vi "S4GUI.vi"(7 "Tab ObsEng":enum32{"Obs", "CCD modes", "Guider", "Eng"}(tab)) -> ()   [LabVIEW 2018] (continued)
                    n4631 = invoke class="VI" method="Run VI"(reference=w10986, error in=w10987, "Wait until done"=w10984, "Auto Dispose Ref"=w10984) -> ()  [unwired: 1 in, 5 out]
                  }
                }
              }
            }
            n4632 = Number To Decimal String(number="Target Temp 4") -> (decimal integer string=w10906:string)  [unwired: 1 in]
            n4633 = call-dynamic "Write Channel.vi"("error in (no error)"=w10889, "Channel.lvclass"=w10892, "Acquisition in"=w10891) -> ("error out"=w10922:errorcluster, "Acquisition out"=w10923:refnum<class "Acquisition.lvclass">)  [unwired: 7 in]
            n4634 = Concatenate Strings("SET TEMP [" ("User Event"), w10906, "] CLICKED - CH4" ("User Event")) -> (w10905:string)
            n4635 = call-dynamic "Write AcquisitionD.vi"("error in (no error)"=w10922, "Acquisition.lvclass"=w10923, "S4ACS_GUI in"=w10890) -> ("error out"=w10900:errorcluster, "S4ACS_GUI out"=w10901:refnum<class "S4GUI.lvclass">)  [unwired: 7 in]
            n4636 = call-dynamic "Write User Event.vi"("error in (no error)"=w10900, "User Event"=w10905, "S4GUI in"=w10901) -> ("error out"=w10898:errorcluster, "S4GUI out"=w10899:refnum<class "S4GUI.lvclass">)  [unwired: 7 in]
          }
        }
      }
      event "SET Temp message": Value Change {
        # "Seleção do modo de apresentação da\nmensagem de erro para o SET de \ntemperatura manual:\nF: via Last Error em vermelho (S4GUI:HandleObservation.vi);\nT: via janela de popup (MsgTempPopup.vi)."
        n4637 = event-data() -> ("NewVal"=w10993:bool)  [unwired: 1 in]
        n4638 = call-dynamic "Write SET temp error mode.vi"("error in (no error)"=w10994, "SET temp error mode"=w10993, "S4GUI in"=w10995) -> ("error out"=w10991:errorcluster, "S4GUI out"=w10992:refnum<class "S4GUI.lvclass">)  [unwired: 7 in]
      }
      event "Avança Estado": Value Change {
        n4639 = event-data() -> ()  [unwired: 1 in, 4 out]
        n4640 = call-dynamic "Read Sync Box.lvclass.vi"("error in (no error)"=w11004, "SPARC4_AC in"=w11005) -> ("error out"=w11017:errorcluster, "Sync Box.lvclass"=w11018:refnum<class "Sync Box.lvclass">, "SPARC4_AC out"=w11009:refnum<class "S4GUI.lvclass">)  [unwired: 7 in]
        n4641 = call-dynamic "Read Trigger.lvclass.vi"("error in (no error)"=w11017, "Sync Box in"=w11018) -> ("error out"=w11015:errorcluster, "Trigger.lvclass"=w11016:refnum<class "Trigger.lvclass">, "Sync Box out"=w11012:refnum<class "Sync Box.lvclass">)  [unwired: 7 in]
        n4642 = call-dynamic "Read State Machine.vi"("error in (no error)"=w11015, "Device in"=w11016) -> ("error out"=w11001:errorcluster, "State Machine.lvclass"=w11002:refnum<class "State Machine.lvclass">, "Device out"=w11013:refnum<class "Trigger.lvclass">)  [unwired: 7 in]
        n4643 = call-dynamic "Read State.vi"("error in (no error)"=w11001, "State Machine in"=w11002) -> ("error out"=w10997:errorcluster, "State"=w11000:i32, "State Machine out"=w10998:refnum<class "State Machine.lvclass">)  [unwired: 7 in]
        n4644 = Increment(x=w11000) -> (x+1=w10999:i32)
        n4645 = call "Next State.vi"("error in (no error)"=w10997, "New_State"=w10999, "State Machine in"=w10998) -> ("error out"=w11011:errorcluster, "State Machine out"=w11014:refnum<class "State Machine.lvclass">)  [unwired: 7 in]
        n4646 = call-dynamic "Write State Machine.vi"("error in (no error)"=w11011, "State Machine.lvclass"=w11014, "Device in"=w11013) -> ("error out"=w11007:errorcluster, "Device out"=w11006:refnum<class "Trigger.lvclass">)  [unwired: 7 in]
        n4647 = call-dynamic "Write Trigger.lvclass.vi"("error in (no error)"=w11007, "Trigger.lvclass"=w11006, "Sync Box in"=w11012) -> ("error out"=w11008:errorcluster, "Sync Box out"=w11010:refnum<class "Sync Box.lvclass">)  [unwired: 7 in]
        n4648 = call-dynamic "Write Sync Box.lvclass.vi"("error in (no error)"=w11008, "Sync Box.lvclass"=w11010, "SPARC4_AC in"=w11009) -> ("error out"=w11003:errorcluster, "SPARC4_AC out"=w10996:refnum<class "S4GUI.lvclass">)  [unwired: 7 in]
      }
      event "DelayA": Value Change {
        n4649 = event-data() -> ("NewVal"=w11020:string)  [unwired: 1 in, 3 out]
        n4650 = call-dynamic "Read Sync Box.lvclass.vi"("error in (no error)"=w11024, "SPARC4_AC in"=w11025) -> ("error out"=w11032:errorcluster, "Sync Box.lvclass"=w11033:refnum<class "Sync Box.lvclass">, "SPARC4_AC out"=w11029:refnum<class "S4GUI.lvclass">)  [unwired: 7 in]
        n4651 = call-dynamic "Read Trigger.lvclass.vi"("error in (no error)"=w11032, "Sync Box in"=w11033) -> ("error out"=w11021:errorcluster, "Trigger.lvclass"=w11022:refnum<class "Trigger.lvclass">, "Sync Box out"=w11031:refnum<class "Sync Box.lvclass">)  [unwired: 7 in]
        n4652 = call-dynamic "Write DelayA.vi"("error in (no error)"=w11021, "DelayA"=w11020, "Trigger in"=w11022) -> ("error out"=w11027:errorcluster, "Trigger out"=w11026:refnum<class "Trigger.lvclass">)  [unwired: 7 in]
        n4653 = call-dynamic "Write Trigger.lvclass.vi"("error in (no error)"=w11027, "Trigger.lvclass"=w11026, "Sync Box in"=w11031) -> ("error out"=w11028:errorcluster, "Sync Box out"=w11030:refnum<class "Sync Box.lvclass">)  [unwired: 7 in]
        n4654 = call-dynamic "Write Sync Box.lvclass.vi"("error in (no error)"=w11028, "Sync Box.lvclass"=w11030, "SPARC4_AC in"=w11029) -> ("error out"=w11023:errorcluster, "SPARC4_AC out"=w11019:refnum<class "S4GUI.lvclass">)  [unwired: 7 in]
      }
      event "DelayB": Value Change {
        n4655 = event-data() -> ("NewVal"=w11035:string)  [unwired: 1 in, 3 out]
        n4656 = call-dynamic "Read Sync Box.lvclass.vi"("error in (no error)"=w11039, "SPARC4_AC in"=w11040) -> ("error out"=w11047:errorcluster, "Sync Box.lvclass"=w11048:refnum<class "Sync Box.lvclass">, "SPARC4_AC out"=w11044:refnum<class "S4GUI.lvclass">)  [unwired: 7 in]
        n4657 = call-dynamic "Read Trigger.lvclass.vi"("error in (no error)"=w11047, "Sync Box in"=w11048) -> ("error out"=w11036:errorcluster, "Trigger.lvclass"=w11037:refnum<class "Trigger.lvclass">, "Sync Box out"=w11046:refnum<class "Sync Box.lvclass">)  [unwired: 7 in]
        n4658 = call-dynamic "Write DelayB.vi"("error in (no error)"=w11036, "DelayB"=w11035, "Trigger in"=w11037) -> ("error out"=w11042:errorcluster, "Trigger out"=w11041:refnum<class "Trigger.lvclass">)  [unwired: 7 in]
        n4659 = call-dynamic "Write Trigger.lvclass.vi"("error in (no error)"=w11042, "Trigger.lvclass"=w11041, "Sync Box in"=w11046) -> ("error out"=w11043:errorcluster, "Sync Box out"=w11045:refnum<class "Sync Box.lvclass">)  [unwired: 7 in]
        n4660 = call-dynamic "Write Sync Box.lvclass.vi"("error in (no error)"=w11043, "Sync Box.lvclass"=w11045, "SPARC4_AC in"=w11044) -> ("error out"=w11038:errorcluster, "SPARC4_AC out"=w11034:refnum<class "S4GUI.lvclass">)  [unwired: 7 in]
      }
      event "DelayC": Value Change {
        n4661 = event-data() -> ("NewVal"=w11050:string)  [unwired: 1 in, 3 out]
        n4662 = call-dynamic "Read Sync Box.lvclass.vi"("error in (no error)"=w11054, "SPARC4_AC in"=w11055) -> ("error out"=w11062:errorcluster, "Sync Box.lvclass"=w11063:refnum<class "Sync Box.lvclass">, "SPARC4_AC out"=w11059:refnum<class "S4GUI.lvclass">)  [unwired: 7 in]
        n4663 = call-dynamic "Read Trigger.lvclass.vi"("error in (no error)"=w11062, "Sync Box in"=w11063) -> ("error out"=w11051:errorcluster, "Trigger.lvclass"=w11052:refnum<class "Trigger.lvclass">, "Sync Box out"=w11061:refnum<class "Sync Box.lvclass">)  [unwired: 7 in]
        n4664 = call-dynamic "Write DelayC.vi"("error in (no error)"=w11051, "DelayC"=w11050, "Trigger in"=w11052) -> ("error out"=w11057:errorcluster, "Trigger out"=w11056:refnum<class "Trigger.lvclass">)  [unwired: 7 in]
        n4665 = call-dynamic "Write Trigger.lvclass.vi"("error in (no error)"=w11057, "Trigger.lvclass"=w11056, "Sync Box in"=w11061) -> ("error out"=w11058:errorcluster, "Sync Box out"=w11060:refnum<class "Sync Box.lvclass">)  [unwired: 7 in]
        n4666 = call-dynamic "Write Sync Box.lvclass.vi"("error in (no error)"=w11058, "Sync Box.lvclass"=w11060, "SPARC4_AC in"=w11059) -> ("error out"=w11053:errorcluster, "SPARC4_AC out"=w11049:refnum<class "S4GUI.lvclass">)  [unwired: 7 in]
      }
      event "DelayD": Value Change {
        n4667 = event-data() -> ("NewVal"=w11065:string)  [unwired: 1 in, 3 out]
        n4668 = call-dynamic "Read Sync Box.lvclass.vi"("error in (no error)"=w11069, "SPARC4_AC in"=w11070) -> ("error out"=w11077:errorcluster, "Sync Box.lvclass"=w11078:refnum<class "Sync Box.lvclass">, "SPARC4_AC out"=w11074:refnum<class "S4GUI.lvclass">)  [unwired: 7 in]
        n4669 = call-dynamic "Read Trigger.lvclass.vi"("error in (no error)"=w11077, "Sync Box in"=w11078) -> ("error out"=w11066:errorcluster, "Trigger.lvclass"=w11067:refnum<class "Trigger.lvclass">, "Sync Box out"=w11076:refnum<class "Sync Box.lvclass">)  [unwired: 7 in]
        n4670 = call-dynamic "Write DelayD.vi"("error in (no error)"=w11066, "DelayD"=w11065, "Trigger in"=w11067) -> ("error out"=w11072:errorcluster, "Trigger out"=w11071:refnum<class "Trigger.lvclass">)  [unwired: 7 in]
        n4671 = call-dynamic "Write Trigger.lvclass.vi"("error in (no error)"=w11072, "Trigger.lvclass"=w11071, "Sync Box in"=w11076) -> ("error out"=w11073:errorcluster, "Sync Box out"=w11075:refnum<class "Sync Box.lvclass">)  [unwired: 7 in]
        n4672 = call-dynamic "Write Sync Box.lvclass.vi"("error in (no error)"=w11073, "Sync Box.lvclass"=w11075, "SPARC4_AC in"=w11074) -> ("error out"=w11068:errorcluster, "SPARC4_AC out"=w11064:refnum<class "S4GUI.lvclass">)  [unwired: 7 in]
      }
      event "WidthA": Value Change {
        n4673 = event-data() -> ("NewVal"=w11080:string)  [unwired: 1 in, 3 out]
        n4674 = call-dynamic "Read Sync Box.lvclass.vi"("error in (no error)"=w11084, "SPARC4_AC in"=w11085) -> ("error out"=w11092:errorcluster, "Sync Box.lvclass"=w11093:refnum<class "Sync Box.lvclass">, "SPARC4_AC out"=w11089:refnum<class "S4GUI.lvclass">)  [unwired: 7 in]
        n4675 = call-dynamic "Read Trigger.lvclass.vi"("error in (no error)"=w11092, "Sync Box in"=w11093) -> ("error out"=w11081:errorcluster, "Trigger.lvclass"=w11082:refnum<class "Trigger.lvclass">, "Sync Box out"=w11091:refnum<class "Sync Box.lvclass">)  [unwired: 7 in]
        n4676 = call-dynamic "Write WidthA.vi"("error in (no error)"=w11081, "WidthA"=w11080, "Trigger in"=w11082) -> ("error out"=w11087:errorcluster, "Trigger out"=w11086:refnum<class "Trigger.lvclass">)  [unwired: 7 in]
        n4677 = call-dynamic "Write Trigger.lvclass.vi"("error in (no error)"=w11087, "Trigger.lvclass"=w11086, "Sync Box in"=w11091) -> ("error out"=w11088:errorcluster, "Sync Box out"=w11090:refnum<class "Sync Box.lvclass">)  [unwired: 7 in]
        n4678 = call-dynamic "Write Sync Box.lvclass.vi"("error in (no error)"=w11088, "Sync Box.lvclass"=w11090, "SPARC4_AC in"=w11089) -> ("error out"=w11083:errorcluster, "SPARC4_AC out"=w11079:refnum<class "S4GUI.lvclass">)  [unwired: 7 in]
      }
      event "WidthB": Value Change {
        n4679 = event-data() -> ("NewVal"=w11095:string)  [unwired: 1 in, 3 out]
        n4680 = call-dynamic "Read Sync Box.lvclass.vi"("error in (no error)"=w11099, "SPARC4_AC in"=w11100) -> ("error out"=w11107:errorcluster, "Sync Box.lvclass"=w11108:refnum<class "Sync Box.lvclass">, "SPARC4_AC out"=w11104:refnum<class "S4GUI.lvclass">)  [unwired: 7 in]
        n4681 = call-dynamic "Read Trigger.lvclass.vi"("error in (no error)"=w11107, "Sync Box in"=w11108) -> ("error out"=w11096:errorcluster, "Trigger.lvclass"=w11097:refnum<class "Trigger.lvclass">, "Sync Box out"=w11106:refnum<class "Sync Box.lvclass">)  [unwired: 7 in]
        n4682 = call-dynamic "Write WidthB.vi"("error in (no error)"=w11096, "WidthB"=w11095, "Trigger in"=w11097) -> ("error out"=w11102:errorcluster, "Trigger out"=w11101:refnum<class "Trigger.lvclass">)  [unwired: 7 in]
        n4683 = call-dynamic "Write Trigger.lvclass.vi"("error in (no error)"=w11102, "Trigger.lvclass"=w11101, "Sync Box in"=w11106) -> ("error out"=w11103:errorcluster, "Sync Box out"=w11105:refnum<class "Sync Box.lvclass">)  [unwired: 7 in]
        n4684 = call-dynamic "Write Sync Box.lvclass.vi"("error in (no error)"=w11103, "Sync Box.lvclass"=w11105, "SPARC4_AC in"=w11104) -> ("error out"=w11098:errorcluster, "SPARC4_AC out"=w11094:refnum<class "S4GUI.lvclass">)  [unwired: 7 in]
      }
      event "WidthC": Value Change {
        n4685 = event-data() -> ("NewVal"=w11110:string)  [unwired: 1 in, 3 out]
        n4686 = call-dynamic "Read Sync Box.lvclass.vi"("error in (no error)"=w11114, "SPARC4_AC in"=w11115) -> ("error out"=w11122:errorcluster, "Sync Box.lvclass"=w11123:refnum<class "Sync Box.lvclass">, "SPARC4_AC out"=w11119:refnum<class "S4GUI.lvclass">)  [unwired: 7 in]
        n4687 = call-dynamic "Read Trigger.lvclass.vi"("error in (no error)"=w11122, "Sync Box in"=w11123) -> ("error out"=w11111:errorcluster, "Trigger.lvclass"=w11112:refnum<class "Trigger.lvclass">, "Sync Box out"=w11121:refnum<class "Sync Box.lvclass">)  [unwired: 7 in]
        n4688 = call-dynamic "Write WidthC.vi"("error in (no error)"=w11111, "WidthC"=w11110, "Trigger in"=w11112) -> ("error out"=w11117:errorcluster, "Trigger out"=w11116:refnum<class "Trigger.lvclass">)  [unwired: 7 in]
        n4689 = call-dynamic "Write Trigger.lvclass.vi"("error in (no error)"=w11117, "Trigger.lvclass"=w11116, "Sync Box in"=w11121) -> ("error out"=w11118:errorcluster, "Sync Box out"=w11120:refnum<class "Sync Box.lvclass">)  [unwired: 7 in]
        n4690 = call-dynamic "Write Sync Box.lvclass.vi"("error in (no error)"=w11118, "Sync Box.lvclass"=w11120, "SPARC4_AC in"=w11119) -> ("error out"=w11113:errorcluster, "SPARC4_AC out"=w11109:refnum<class "S4GUI.lvclass">)  [unwired: 7 in]
      }
      event "WidthD": Value Change {
        n4691 = event-data() -> ("NewVal"=w11125:string)  [unwired: 1 in, 3 out]
        n4692 = call-dynamic "Read Sync Box.lvclass.vi"("error in (no error)"=w11129, "SPARC4_AC in"=w11130) -> ("error out"=w11137:errorcluster, "Sync Box.lvclass"=w11138:refnum<class "Sync Box.lvclass">, "SPARC4_AC out"=w11134:refnum<class "S4GUI.lvclass">)  [unwired: 7 in]
        n4693 = call-dynamic "Read Trigger.lvclass.vi"("error in (no error)"=w11137, "Sync Box in"=w11138) -> ("error out"=w11126:errorcluster, "Trigger.lvclass"=w11127:refnum<class "Trigger.lvclass">, "Sync Box out"=w11136:refnum<class "Sync Box.lvclass">)  [unwired: 7 in]
        n4694 = call-dynamic "Write WidthD.vi"("error in (no error)"=w11126, "WidthD"=w11125, "Trigger in"=w11127) -> ("error out"=w11132:errorcluster, "Trigger out"=w11131:refnum<class "Trigger.lvclass">)  [unwired: 7 in]
        n4695 = call-dynamic "Write Trigger.lvclass.vi"("error in (no error)"=w11132, "Trigger.lvclass"=w11131, "Sync Box in"=w11136) -> ("error out"=w11133:errorcluster, "Sync Box out"=w11135:refnum<class "Sync Box.lvclass">)  [unwired: 7 in]
        n4696 = call-dynamic "Write Sync Box.lvclass.vi"("error in (no error)"=w11133, "Sync Box.lvclass"=w11135, "SPARC4_AC in"=w11134) -> ("error out"=w11128:errorcluster, "SPARC4_AC out"=w11124:refnum<class "S4GUI.lvclass">)  [unwired: 7 in]
      }
      event "WPROT_set": Value Change {
        # "Espera até 10 x 1s = 10s\npara condition de WPROT\n ir para READY"
        n4697 = event-data() -> ()  [unwired: 1 in, 4 out]
        n4698 = call "Read Instrument.lvclass.vi"("error in (no error)"=w11160, "S4ACS_GUI in"=w11161) -> ("error out"=w11158:errorcluster, "Instrument.lvclass"=w11159:refnum<class "Instrument.lvclass">, "S4ACS_GUI out"=w11147:refnum<class "S4GUI.lvclass">)  [unwired: 7 in]
        n4699 = call "Read WPROT.vi"("error in (no error)"=w11158, "Instrument in"=w11159) -> ("error out"=w11154:errorcluster, "Opt_Selector.lvclass"=w11157:refnum<class "Opt_Selector.lvclass">, "Instrument out"=w11150:refnum<class "Instrument.lvclass">)  [unwired: 7 in]
        n4700 = call-dynamic "Read State Machine.vi"("error in (no error)"=w11154, "Device in"=w11157) -> ("error out"=w11153:errorcluster, "State Machine.lvclass"=w11156:refnum<class "State Machine.lvclass">, "Device out"=w11152:refnum<class "Opt_Selector.lvclass">)  [unwired: 7 in]
        n4701 = call "Next State.vi"("error in (no error)"=w11153, "New_State"=1, "State Machine in"=w11156) -> ("error out"=w11141:errorcluster, "State Machine out"=w11143:refnum<class "State Machine.lvclass">)  [unwired: 7 in]
        n4702 = call-dynamic "Write Timer.vi"("error in (no error)"=w11141, "Timer"=u32 10, "State Machine in"=w11143) -> ("error out"=w11140:errorcluster, "State Machine out"=w11142:refnum<class "State Machine.lvclass">)  [unwired: 7 in]
        n4703 = call-dynamic "Write State Machine.vi"("error in (no error)"=w11140, "State Machine.lvclass"=w11142, "Device in"=w11152) -> ("error out"=w11149:errorcluster, "Device out"=w11151:refnum<class "Opt_Selector.lvclass">)  [unwired: 7 in]
        n4704 = call "Write WPROT.vi"("error in (no error)"=w11149, "Opt_Selector.lvclass"=w11151, "Instrument in"=w11150) -> ("error out"=w11146:errorcluster, "Instrument out"=w11148:refnum<class "Instrument.lvclass">)  [unwired: 7 in]
        n4705 = call "Write Instrument.lvclass.vi"("error in (no error)"=w11146, "Instrument.lvclass"=w11148, "S4ACS_GUI in"=w11147) -> ("error out"=w11145:errorcluster, "S4ACS_GUI out"=w11144:refnum<class "S4GUI.lvclass">)  [unwired: 7 in]
      }
      event "TARGET NAME WPROT": Value Change {
        n4706 = event-data() -> ()  [unwired: 1 in, 1 out]
        n4707 = call "Read Instrument.lvclass.vi"("error in (no error)"=w11189, "S4ACS_GUI in"=w11190) -> ("error out"=w11197:errorcluster, "Instrument.lvclass"=w11198:refnum<class "Instrument.lvclass">, "S4ACS_GUI out"=w11192:refnum<class "S4GUI.lvclass">)  [unwired: 7 in]
        n4708 = property on="TARGET NAME WPROT" class="Enum (strict)"() -> ("RingText.Text"=w11188:string)  [unwired: 2 in, 2 out]
        n4709 = Build Array(-1.0 ("element"), 0.0 ("element"), 22.5 ("element"), 45.0 ("element"), 67.5 ("element"), 90.0 ("element"), 112.5 ("element"), 135.0 ("element"), 157.5 ("element"), 180.0 ("element"), 202.5 ("element"), 225.0 ("element"), 247.5 ("element"), 270.0 ("element"), 292.5 ("element"), 315.0 ("element"), 337.5 ("element")) -> (w11180:dbl[])
        n4710 = call "Read WPROT.vi"("error in (no error)"=w11197, "Instrument in"=w11198) -> ("error out"=w11195:errorcluster, "Opt_Selector.lvclass"=w11196:refnum<class "Opt_Selector.lvclass">, "Instrument out"=w11194:refnum<class "Instrument.lvclass">)  [unwired: 7 in]
        n4711 = call "Write target name.vi"("error in (no error)"=w11195, "target name"=w11188, "Optics in"=w11196) -> ("error out"=w11176:errorcluster, "Optics out"=w11177:refnum<class "Opt_Selector.lvclass">)  [unwired: 7 in]
        n4712 = Index Array(array=w11180, index="TARGET NAME WPROT") -> (element=w11178:dbl)
        n4713 = call "Write target.vi"("error in (no error)"=w11176, "target"=w11178, "Optics in"=w11177) -> ("error out"=w11175:errorcluster, "Optics out"=w11174:refnum<class "Opt_Selector.lvclass">)  [unwired: 7 in]
        n4714 = call "Write WPROT.vi"("error in (no error)"=w11175, "Opt_Selector.lvclass"=w11174, "Instrument in"=w11194) -> ("error out"=w11191:errorcluster, "Instrument out"=w11193:refnum<class "Instrument.lvclass">)  [unwired: 7 in]
        n4715 = call "Write Instrument.lvclass.vi"("error in (no error)"=w11191, "Instrument.lvclass"=w11193, "S4ACS_GUI in"=w11192) -> ("error out"=w11187:errorcluster, "S4ACS_GUI out"=w11162:refnum<class "S4GUI.lvclass">)  [unwired: 7 in]
      }
      event "TARGET NAME WPSEL": Value Change {
        n4716 = event-data() -> ()  [unwired: 1 in, 1 out]
        n4717 = call "Read Instrument.lvclass.vi"("error in (no error)"=w11213, "S4ACS_GUI in"=w11214) -> ("error out"=w11221:errorcluster, "Instrument.lvclass"=w11222:refnum<class "Instrument.lvclass">, "S4ACS_GUI out"=w11216:refnum<class "S4GUI.lvclass">)  [unwired: 7 in]
        n4718 = property on="TARGET NAME WPSEL" class="Enum (strict)"() -> ("RingText.Text"=w11200:string)  [unwired: 2 in, 2 out]
        n4719 = Build Array(-1.0 ("element"), 80.0 ("element"), 0.0 ("element"), 160.0 ("element")) -> (w11207:dbl[])
        n4720 = call "Read WPSEL.vi"("error in (no error)"=w11221, "Instrument in"=w11222) -> ("error out"=w11219:errorcluster, "Opt_Selector.lvclass"=w11220:refnum<class "Opt_Selector.lvclass">, "Instrument out"=w11218:refnum<class "Instrument.lvclass">)  [unwired: 7 in]
        n4721 = call "Write target name.vi"("error in (no error)"=w11219, "target name"=w11200, "Optics in"=w11220) -> ("error out"=w11204:errorcluster, "Optics out"=w11205:refnum<class "Opt_Selector.lvclass">)  [unwired: 7 in]
        n4722 = Index Array(array=w11207, index="TARGET NAME WPSEL") -> (element=w11206:dbl)
        n4723 = call "Write target.vi"("error in (no error)"=w11204, "target"=w11206, "Optics in"=w11205) -> ("error out"=w11203:errorcluster, "Optics out"=w11202:refnum<class "Opt_Selector.lvclass">)  [unwired: 7 in]
        n4724 = call "Write WPSEL.vi"("error in (no error)"=w11203, "Opt_Selector.lvclass"=w11202, "Instrument in"=w11218) -> ("error out"=w11215:errorcluster, "Instrument out"=w11217:refnum<class "Instrument.lvclass">)  [unwired: 7 in]
        n4725 = call "Write Instrument.lvclass.vi"("error in (no error)"=w11215, "Instrument.lvclass"=w11217, "S4ACS_GUI in"=w11216) -> ("error out"=w11212:errorcluster, "S4ACS_GUI out"=w11199:refnum<class "S4GUI.lvclass">)  [unwired: 7 in]
      }
      event "Lambda Selector": Value Change {
        n4726 = event-data() -> ("NewVal"=w11224:u16)  [unwired: 1 in, 1 out]
        n4727 = call "Read Instrument.lvclass.vi"("error in (no error)"=w11255, "S4ACS_GUI in"=w11256) -> ("error out"=w11257:errorcluster, "Instrument.lvclass"=w11232:refnum<class "Instrument.lvclass">, "S4ACS_GUI out"=w11229:refnum<class "S4GUI.lvclass">)  [unwired: 7 in]
        n4728 = Build Array(80.0 ("element"), 0.0 ("element"), 160.0 ("element")) -> (w11250:dbl[])
        n4729 = property on="Lambda Selector" class="Ring (strict)"() -> ("RingText.Text"=w11230:string)  [unwired: 2 in, 2 out]
        n4730 = call "Read WPSEL.vi"("error in (no error)"=w11257, "Instrument in"=w11232) -> ("error out"=w11239:errorcluster, "Opt_Selector.lvclass"=w11238:refnum<class "Opt_Selector.lvclass">, "Instrument out"=w11231:refnum<class "Instrument.lvclass">)  [unwired: 7 in]
        n4731 = Index Array(array=w11250, index=w11224) -> (element=w11249:dbl)
        n4732 = call "Write target.vi"("error in (no error)"=w11239, "target"=w11249, "Optics in"=w11238) -> ("error out"=w11236:errorcluster, "Optics out"=w11237:refnum<class "Opt_Selector.lvclass">)  [unwired: 7 in]
        n4733 = case shown="\"OFF\", Default" w11230 {
          selector: w11230 -> [w11260 _ _]
          tunnel: [w11260 "ON" "ON"] -> w11241
          tunnel: [0.0 ("element") 30.0 ("element") 30.0 ("element")] -> w11240
          tunnel: [w11260 "L/2" "L/4"] -> w11233
          frame "OFF", Default {
            n4734 = property on="Calibrator Selector" class="Ring (strict)"("DisabledEnum"=T12."Disabled and Grayed Out" ("Disabled")) -> ()  [unwired: 2 in, 2 out]
          }
          frame "Lambda/2" {
            n4735 = property on="Calibrator Selector" class="Ring (strict)"("DisabledEnum"=T12."Enabled" ("Disabled")) -> ()  [unwired: 2 in, 2 out]
          }
          frame "Lambda/4" {
            n4736 = property on="Calibrator Selector" class="Ring (strict)"("DisabledEnum"=T12."Enabled" ("Disabled")) -> ()  [unwired: 2 in, 2 out]
          }
        }
        n4737 = call "Write target name.vi"("error in (no error)"=w11236, "target name"=w11233, "Optics in"=w11237) -> ("error out"=w11235:errorcluster, "Optics out"=w11234:refnum<class "Opt_Selector.lvclass">)  [unwired: 7 in]
        n4738 = call "Write WPSEL.vi"("error in (no error)"=w11235, "Opt_Selector.lvclass"=w11234, "Instrument in"=w11231) -> ("error out"=w11226:errorcluster, "Instrument out"=w11225:refnum<class "Instrument.lvclass">)  [unwired: 7 in]
        n4739 = call "Read ASEL.vi"("error in (no error)"=w11226, "Instrument in"=w11225) -> ("error out"=w11246:errorcluster, "Opt_Selector.lvclass"=w11244:refnum<class "Opt_Selector.lvclass">, "Instrument out"=w11228:refnum<class "Instrument.lvclass">)  [unwired: 7 in]
        n4740 = call "Write target name.vi"("error in (no error)"=w11246, "target name"=w11241, "Optics in"=w11244) -> ("error out"=w11247:errorcluster, "Optics out"=w11243:refnum<class "Opt_Selector.lvclass">)  [unwired: 7 in]
        n4741 = call "Write target.vi"("error in (no error)"=w11247, "target"=w11240, "Optics in"=w11243) -> ("error out"=w11248:errorcluster, "Optics out"=w11242:refnum<class "Opt_Selector.lvclass">)  [unwired: 7 in]
        n4742 = call "Write ASEL.vi"("error in (no error)"=w11248, "Opt_Selector.lvclass"=w11242, "Instrument in"=w11228) -> ("error out"=w11245:errorcluster, "Instrument out"=w11227:refnum<class "Instrument.lvclass">)  [unwired: 7 in]
        n4743 = call "Write Instrument.lvclass.vi"("error in (no error)"=w11245, "Instrument.lvclass"=w11227, "S4ACS_GUI in"=w11229) -> ("error out"=w11254:errorcluster, "S4ACS_GUI out"=w11223:refnum<class "S4GUI.lvclass">)  [unwired: 7 in]
      }
      event "Calibrator Selector": Value Change {
        n4744 = event-data() -> ()  [unwired: 1 in, 6 out]
        n4745 = call "Read Instrument.lvclass.vi"("error in (no error)"=w11289, "S4ACS_GUI in"=w11290) -> ("error out"=w11293:errorcluster, "Instrument.lvclass"=w11294:refnum<class "Instrument.lvclass">, "S4ACS_GUI out"=w11291:refnum<class "S4GUI.lvclass">)  [unwired: 7 in]
        n4746 = Build Array(0.0 ("element"), 72.0 ("element"), 144.0 ("element"), 216.0 ("element"), 288.0 ("element")) -> (w11284:dbl[])
        n4747 = call "Read CALW.vi"("error in (no error)"=w11293, "Instrument in"=w11294) -> ("error out"=w11282:errorcluster, "Opt_Selector.lvclass"=w11281:refnum<class "Opt_Selector.lvclass">, "Instrument out"=w11292:refnum<class "Instrument.lvclass">)  [unwired: 7 in]
        n4748 = Index Array(array=w11284, index="Calibrator Selector") -> (element=w11283:dbl)
        n4749 = call "Write target.vi"("error in (no error)"=w11282, "target"=w11283, "Optics in"=w11281) -> ("error out"=w11279:errorcluster, "Optics out"=w11280:refnum<class "Opt_Selector.lvclass">)  [unwired: 7 in]
        n4750 = property on="Calibrator Selector" class="Ring (strict)"() -> ("RingText.Text"=w11275:string)  [unwired: 2 in, 2 out]
        n4751 = case shown="\"POLARIZER\"" w11275 {
          selector: w11275 -> [_ w11296 w11297 w11298 w11299]
          tunnel: ["OFF" w11296 w11297 w11298 w11299] -> w11276
          frame "OFF", Default {
          }
          frame "POLARIZER" {
          }
          frame "DEPOLARIZER" {
          }
          frame "PINHOLE" {
          }
          frame "SHUTTER" {
          }
        }
        n4752 = call "Write target name.vi"("error in (no error)"=w11279, "target name"=w11276, "Optics in"=w11280) -> ("error out"=w11278:errorcluster, "Optics out"=w11277:refnum<class "Opt_Selector.lvclass">)  [unwired: 7 in]
        n4753 = call "Write CALW.vi"("error in (no error)"=w11278, "Opt_Selector.lvclass"=w11277, "Instrument in"=w11292) -> ("error out"=w11272:errorcluster, "Instrument out"=w11273:refnum<class "Instrument.lvclass">)  [unwired: 7 in]
        n4754 = call "Write Instrument.lvclass.vi"("error in (no error)"=w11272, "Instrument.lvclass"=w11273, "S4ACS_GUI in"=w11291) -> ("error out"=w11288:errorcluster, "S4ACS_GUI out"=w11271:refnum<class "S4GUI.lvclass">)  [unwired: 7 in]
      }
      event "TARGET NAME CALW": Value Change {
        # "aqui também"
        # "OV20230825: Valores da sequência original"
        n4755 = event-data() -> ()  [unwired: 1 in, 6 out]
        n4756 = call "Read Instrument.lvclass.vi"("error in (no error)"=w11316, "S4ACS_GUI in"=w11317) -> ("error out"=w11324:errorcluster, "Instrument.lvclass"=w11325:refnum<class "Instrument.lvclass">, "S4ACS_GUI out"=w11319:refnum<class "S4GUI.lvclass">)  [unwired: 7 in]
        n4757 = property on="TARGET NAME CALW" class="Enum (strict)"() -> ("RingText.Text"=w11300:string)  [unwired: 2 in, 2 out]
        n4758 = Build Array(-1.0 ("element"), 0.0 ("element"), 72.0 ("element"), 144.0 ("element"), 216.0 ("element"), 288.0 ("element")) -> (w11310:dbl[])
        n4759 = call "Read CALW.vi"("error in (no error)"=w11324, "Instrument in"=w11325) -> ("error out"=w11322:errorcluster, "Opt_Selector.lvclass"=w11323:refnum<class "Opt_Selector.lvclass">, "Instrument out"=w11321:refnum<class "Instrument.lvclass">)  [unwired: 7 in]
        n4760 = call "Write target name.vi"("error in (no error)"=w11322, "target name"=w11300, "Optics in"=w11323) -> ("error out"=w11307:errorcluster, "Optics out"=w11308:refnum<class "Opt_Selector.lvclass">)  [unwired: 7 in]
        n4761 = Index Array(array=w11310, index="TARGET NAME CALW") -> (element=w11309:dbl)
        n4762 = call "Write target.vi"("error in (no error)"=w11307, "target"=w11309, "Optics in"=w11308) -> ("error out"=w11306:errorcluster, "Optics out"=w11305:refnum<class "Opt_Selector.lvclass">)  [unwired: 7 in]
        n4763 = call "Write CALW.vi"("error in (no error)"=w11306, "Opt_Selector.lvclass"=w11305, "Instrument in"=w11321) -> ("error out"=w11318:errorcluster, "Instrument out"=w11320:refnum<class "Instrument.lvclass">)  [unwired: 7 in]
        n4764 = call "Write Instrument.lvclass.vi"("error in (no error)"=w11318, "Instrument.lvclass"=w11320, "S4ACS_GUI in"=w11319) -> ("error out"=w11315:errorcluster, "S4ACS_GUI out"=w11301:refnum<class "S4GUI.lvclass">)  [unwired: 7 in]
      }
      event "TARGET NAME ASEL": Value Change {
        n4765 = event-data() -> ()  [unwired: 1 in, 6 out]
        n4766 = call "Read Instrument.lvclass.vi"("error in (no error)"=w11339, "S4ACS_GUI in"=w11340) -> ("error out"=w11347:errorcluster, "Instrument.lvclass"=w11348:refnum<class "Instrument.lvclass">, "S4ACS_GUI out"=w11342:refnum<class "S4GUI.lvclass">)  [unwired: 7 in]
        n4767 = Build Array(-1.0 ("element"), 0.0 ("element"), 30.0 ("element")) -> (w11334:dbl[])
        n4768 = call "Read ASEL.vi"("error in (no error)"=w11347, "Instrument in"=w11348) -> ("error out"=w11345:errorcluster, "Opt_Selector.lvclass"=w11346:refnum<class "Opt_Selector.lvclass">, "Instrument out"=w11344:refnum<class "Instrument.lvclass">)  [unwired: 7 in]
        n4769 = property on="TARGET NAME ASEL" class="Enum (strict)"() -> ("RingText.Text"=w11328:string)  [unwired: 2 in, 2 out]
        n4770 = call "Write target name.vi"("error in (no error)"=w11345, "target name"=w11328, "Optics in"=w11346) -> ("error out"=w11331:errorcluster, "Optics out"=w11332:refnum<class "Opt_Selector.lvclass">)  [unwired: 7 in]
        n4771 = Index Array(array=w11334, index="TARGET NAME ASEL") -> (element=w11333:dbl)
        n4772 = call "Write target.vi"("error in (no error)"=w11331, "target"=w11333, "Optics in"=w11332) -> ("error out"=w11330:errorcluster, "Optics out"=w11329:refnum<class "Opt_Selector.lvclass">)  [unwired: 7 in]
        n4773 = call "Write ASEL.vi"("error in (no error)"=w11330, "Opt_Selector.lvclass"=w11329, "Instrument in"=w11344) -> ("error out"=w11341:errorcluster, "Instrument out"=w11343:refnum<class "Instrument.lvclass">)  [unwired: 7 in]
        n4774 = call "Write Instrument.lvclass.vi"("error in (no error)"=w11341, "Instrument.lvclass"=w11343, "S4ACS_GUI in"=w11342) -> ("error out"=w11338:errorcluster, "S4ACS_GUI out"=w11326:refnum<class "S4GUI.lvclass">)  [unwired: 7 in]
      }
      event "WPROT_stop": Value Change {
        n4775 = event-data() -> ()  [unwired: 1 in, 4 out]
        n4776 = call "Read Instrument.lvclass.vi"("error in (no error)"=w11367, "S4ACS_GUI in"=w11368) -> ("error out"=w11365:errorcluster, "Instrument.lvclass"=w11366:refnum<class "Instrument.lvclass">, "S4ACS_GUI out"=w11352:refnum<class "S4GUI.lvclass">)  [unwired: 7 in]
        n4777 = call "Read WPROT.vi"("error in (no error)"=w11365, "Instrument in"=w11366) -> ("error out"=w11361:errorcluster, "Opt_Selector.lvclass"=w11364:refnum<class "Opt_Selector.lvclass">, "Instrument out"=w11355:refnum<class "Instrument.lvclass">)  [unwired: 7 in]
        n4778 = call-dynamic "Read State Machine.vi"("error in (no error)"=w11361, "Device in"=w11364) -> ("error out"=w11360:errorcluster, "State Machine.lvclass"=w11363:refnum<class "State Machine.lvclass">, "Device out"=w11357:refnum<class "Opt_Selector.lvclass">)  [unwired: 7 in]
        n4779 = call "Next State.vi"("error in (no error)"=w11360, "New_State"=10, "State Machine in"=w11363) -> ("error out"=w11359:errorcluster, "State Machine out"=w11358:refnum<class "State Machine.lvclass">)  [unwired: 7 in]
        n4780 = call-dynamic "Write State Machine.vi"("error in (no error)"=w11359, "State Machine.lvclass"=w11358, "Device in"=w11357) -> ("error out"=w11354:errorcluster, "Device out"=w11356:refnum<class "Opt_Selector.lvclass">)  [unwired: 7 in]
        n4781 = call "Write WPROT.vi"("error in (no error)"=w11354, "Opt_Selector.lvclass"=w11356, "Instrument in"=w11355) -> ("error out"=w11351:errorcluster, "Instrument out"=w11353:refnum<class "Instrument.lvclass">)  [unwired: 7 in]
        n4782 = call "Write Instrument.lvclass.vi"("error in (no error)"=w11351, "Instrument.lvclass"=w11353, "S4ACS_GUI in"=w11352) -> ("error out"=w11350:errorcluster, "S4ACS_GUI out"=w11349:refnum<class "S4GUI.lvclass">)  [unwired: 7 in]
      }
      event "WPROT_init": Value Change {
        n4783 = event-data() -> ()  [unwired: 1 in, 4 out]
        n4784 = call "Read Instrument.lvclass.vi"("error in (no error)"=w11387, "S4ACS_GUI in"=w11388) -> ("error out"=w11385:errorcluster, "Instrument.lvclass"=w11386:refnum<class "Instrument.lvclass">, "S4ACS_GUI out"=w11372:refnum<class "S4GUI.lvclass">)  [unwired: 7 in]
        n4785 = call "Read WPROT.vi"("error in (no error)"=w11385, "Instrument in"=w11386) -> ("error out"=w11381:errorcluster, "Opt_Selector.lvclass"=w11384:refnum<class "Opt_Selector.lvclass">, "Instrument out"=w11375:refnum<class "Instrument.lvclass">)  [unwired: 7 in]
        n4786 = call-dynamic "Read State Machine.vi"("error in (no error)"=w11381, "Device in"=w11384) -> ("error out"=w11380:errorcluster, "State Machine.lvclass"=w11383:refnum<class "State Machine.lvclass">, "Device out"=w11377:refnum<class "Opt_Selector.lvclass">)  [unwired: 7 in]
        n4787 = call "Next State.vi"("error in (no error)"=w11380, "New_State"=30, "State Machine in"=w11383) -> ("error out"=w11379:errorcluster, "State Machine out"=w11378:refnum<class "State Machine.lvclass">)  [unwired: 7 in]
        n4788 = call-dynamic "Write State Machine.vi"("error in (no error)"=w11379, "State Machine.lvclass"=w11378, "Device in"=w11377) -> ("error out"=w11374:errorcluster, "Device out"=w11376:refnum<class "Opt_Selector.lvclass">)  [unwired: 7 in]
        n4789 = call "Write WPROT.vi"("error in (no error)"=w11374, "Opt_Selector.lvclass"=w11376, "Instrument in"=w11375) -> ("error out"=w11371:errorcluster, "Instrument out"=w11373:refnum<class "Instrument.lvclass">)  [unwired: 7 in]
        n4790 = call "Write Instrument.lvclass.vi"("error in (no error)"=w11371, "Instrument.lvclass"=w11373, "S4ACS_GUI in"=w11372) -> ("error out"=w11370:errorcluster, "S4ACS_GUI out"=w11369:refnum<class "S4GUI.lvclass">)  [unwired: 7 in]
      }
      event "WPSEL_target": Value Change {
        n4791 = event-data() -> ("NewVal"=w11398:dbl)  [unwired: 1 in, 3 out]
        n4792 = call "Read Instrument.lvclass.vi"("error in (no error)"=w11402, "S4ACS_GUI in"=w11403) -> ("error out"=w11400:errorcluster, "Instrument.lvclass"=w11401:refnum<class "Instrument.lvclass">, "S4ACS_GUI out"=w11392:refnum<class "S4GUI.lvclass">)  [unwired: 7 in]
        n4793 = call "Read WPSEL.vi"("error in (no error)"=w11400, "Instrument in"=w11401) -> ("error out"=w11397:errorcluster, "Opt_Selector.lvclass"=w11399:refnum<class "Opt_Selector.lvclass">, "Instrument out"=w11395:refnum<class "Instrument.lvclass">)  [unwired: 7 in]
        n4794 = call "Write target.vi"("error in (no error)"=w11397, "target"=w11398, "Optics in"=w11399) -> ("error out"=w11394:errorcluster, "Optics out"=w11396:refnum<class "Opt_Selector.lvclass">)  [unwired: 7 in]
        n4795 = call "Write WPSEL.vi"("error in (no error)"=w11394, "Opt_Selector.lvclass"=w11396, "Instrument in"=w11395) -> ("error out"=w11391:errorcluster, "Instrument out"=w11393:refnum<class "Instrument.lvclass">)  [unwired: 7 in]
        n4796 = call "Write Instrument.lvclass.vi"("error in (no error)"=w11391, "Instrument.lvclass"=w11393, "S4ACS_GUI in"=w11392) -> ("error out"=w11390:errorcluster, "S4ACS_GUI out"=w11389:refnum<class "S4GUI.lvclass">)  [unwired: 7 in]
      }
      event "WPSEL_set": Value Change {
        n4797 = event-data() -> ()  [unwired: 1 in, 4 out]
        n4798 = call "Read Instrument.lvclass.vi"("error in (no error)"=w11422, "S4ACS_GUI in"=w11423) -> ("error out"=w11420:errorcluster, "Instrument.lvclass"=w11421:refnum<class "Instrument.lvclass">, "S4ACS_GUI out"=w11408:refnum<class "S4GUI.lvclass">)  [unwired: 7 in]
        n4799 = call "Read WPSEL.vi"("error in (no error)"=w11420, "Instrument in"=w11421) -> ("error out"=w11417:errorcluster, "Opt_Selector.lvclass"=w11419:refnum<class "Opt_Selector.lvclass">, "Instrument out"=w11411:refnum<class "Instrument.lvclass">)  [unwired: 7 in]
        n4800 = call-dynamic "Read State Machine.vi"("error in (no error)"=w11417, "Device in"=w11419) -> ("error out"=w11416:errorcluster, "State Machine.lvclass"=w11405:refnum<class "State Machine.lvclass">, "Device out"=w11413:refnum<class "Opt_Selector.lvclass">)  [unwired: 7 in]
        n4801 = call "Next State.vi"("error in (no error)"=w11416, "New_State"=1, "State Machine in"=w11405) -> ("error out"=w11415:errorcluster, "State Machine out"=w11414:refnum<class "State Machine.lvclass">)  [unwired: 7 in]
        n4802 = call-dynamic "Write State Machine.vi"("error in (no error)"=w11415, "State Machine.lvclass"=w11414, "Device in"=w11413) -> ("error out"=w11410:errorcluster, "Device out"=w11412:refnum<class "Opt_Selector.lvclass">)  [unwired: 7 in]
        n4803 = call "Write WPSEL.vi"("error in (no error)"=w11410, "Opt_Selector.lvclass"=w11412, "Instrument in"=w11411) -> ("error out"=w11407:errorcluster, "Instrument out"=w11409:refnum<class "Instrument.lvclass">)  [unwired: 7 in]
        n4804 = call "Write Instrument.lvclass.vi"("error in (no error)"=w11407, "Instrument.lvclass"=w11409, "S4ACS_GUI in"=w11408) -> ("error out"=w11406:errorcluster, "S4ACS_GUI out"=w11404:refnum<class "S4GUI.lvclass">)  [unwired: 7 in]
      }
      event "Set Waveplate": Value Change {
        # "OV20230825: Sequência de\nvalores originais."
        # "Garantir que, quando em POLARIMETRIA, pelo menos WP1 esteja selecionado."
        n4805 = event-data() -> ()  [unwired: 1 in, 4 out]
        n4806 = local read "Lambda Selector"() -> (w11527:u16)
        n4807 = property on="Calibrator Selector" class="Ring (strict)"() -> ("RingText.Text"=w11508:string)  [unwired: 2 in, 2 out]
        n4808 = call "Read Instrument.lvclass.vi"("error in (no error)"=w11507, "S4ACS_GUI in"=w11506) -> ("error out"=w11525:errorcluster, "Instrument.lvclass"=w11526:refnum<class "Instrument.lvclass">, "S4ACS_GUI out"=w11523:refnum<class "S4GUI.lvclass">)  [unwired: 7 in]
        n4809 = Build Array(0.0 ("element"), 72.0 ("element"), 144.0 ("element"), 216.0 ("element"), 288.0 ("element")) -> (w11519:dbl[])
        n4810 = local read "Calibrator Selector"() -> (w11509:u16)
        n4811 = Build Array(80.0 ("element"), 0.0 ("element"), 160.0 ("element")) -> (w11553:dbl[])
        n4812 = property on="Lambda Selector" class="Ring (strict)"() -> ("RingText.Text"=w11528:string)  [unwired: 2 in, 2 out]
        n4813 = call "Read CALW.vi"("error in (no error)"=w11525, "Instrument in"=w11526) -> ("error out"=w11517:errorcluster, "Opt_Selector.lvclass"=w11516:refnum<class "Opt_Selector.lvclass">, "Instrument out"=w11524:refnum<class "Instrument.lvclass">)  [unwired: 7 in]
        n4814 = Index Array(array=w11519, index=w11509) -> (element=w11518:dbl)
        n4815 = Index Array(array=w11553, index=w11527) -> (element=w11552:dbl)
        n4816 = call "Write target.vi"("error in (no error)"=w11517, "target"=w11518, "Optics in"=w11516) -> ("error out"=w11514:errorcluster, "Optics out"=w11515:refnum<class "Opt_Selector.lvclass">)  [unwired: 7 in]
        n4817 = case shown="\"OFF\", Default" w11508 {
          tunnel: ["OFF" w11782 "PINHOLE" "SHUTTER" w11787] -> w11426
          frame "OFF", Default {
          }
          frame "POLARIZER" {
            n4818 = disable-structure shown="Enabled" {
              disable-tunnel: ["POLARIZER" "DEPOLARIZER"] -> w11782
              frame Enabled {
              }
              frame Disabled {
                # "OV20230426: Montagem do CALW\nestá com POL e DEPOL invertidos"
              }
            }
          }
          frame "PINHOLE" {
          }
          frame "SHUTTER" {
          }
          frame "DEPOLARIZER" {
            n4819 = disable-structure shown="Enabled" {
              disable-tunnel: ["POLARIZER" "DEPOLARIZER"] -> w11787
              frame Disabled {
                # "OV20230426: Montagem do CALW\nestá com POL e DEPOL invertidos"
              }
              frame Enabled {
              }
            }
          }
        }
        n4820 = case shown="\"OFF\", Default" w11528 {
          tunnel: [w11790 "ON" "ON"] -> w11439
          tunnel: [w11791 w11792 w11795] -> w11544
          tunnel: [w11790 "L/2" "L/4"] -> w11424
          tunnel: [w11791 w11792 w11795] -> w11428
          frame "OFF", Default {
            w11790 = "OFF"
            w11791 = 0.0 ("element")
            n4821 = property on="Lambda Selector" class="Ring (strict)"("RingText.Text"=w11790) -> ()  [unwired: 2 in, 2 out]
          }
          frame "Lambda/2" {
            w11792 = 30.0 ("element")
          }
          frame "Lambda/4" {
            w11795 = 30.0 ("element")
          }
        }
        n4822 = call "Write target name.vi"("error in (no error)"=w11514, "target name"=w11426, "Optics in"=w11515) -> ("error out"=w11513:errorcluster, "Optics out"=w11512:refnum<class "Opt_Selector.lvclass">)  [unwired: 7 in]
        n4823 = call "Write CALW.vi"("error in (no error)"=w11513, "Opt_Selector.lvclass"=w11512, "Instrument in"=w11524) -> ("error out"=w11510:errorcluster, "Instrument out"=w11511:refnum<class "Instrument.lvclass">)  [unwired: 7 in]
        n4824 = Equal To 0?(x=w11428) -> (x = 0?=w11429:bool)
        n4825 = call "Write Instrument.lvclass.vi"("error in (no error)"=w11510, "Instrument.lvclass"=w11511, "S4ACS_GUI in"=w11523) -> ("error out"=w11504:errorcluster, "S4ACS_GUI out"=w11505:refnum<class "S4GUI.lvclass">)  [unwired: 7 in]
        n4826 = call "Read Instrument.lvclass.vi"("error in (no error)"=w11504, "S4ACS_GUI in"=w11505) -> ("error out"=w11557:errorcluster, "Instrument.lvclass"=w11537:refnum<class "Instrument.lvclass">, "S4ACS_GUI out"=w11535:refnum<class "S4GUI.lvclass">)  [unwired: 7 in]
        n4827 = call "Read WPSEL.vi"("error in (no error)"=w11557, "Instrument in"=w11537) -> ("error out"=w11543:errorcluster, "Opt_Selector.lvclass"=w11542:refnum<class "Opt_Selector.lvclass">, "Instrument out"=w11536:refnum<class "Instrument.lvclass">)  [unwired: 7 in]
        n4828 = call "Write target.vi"("error in (no error)"=w11543, "target"=w11552, "Optics in"=w11542) -> ("error out"=w11540:errorcluster, "Optics out"=w11541:refnum<class "Opt_Selector.lvclass">)  [unwired: 7 in]
        n4829 = call "Write target name.vi"("error in (no error)"=w11540, "target name"=w11424, "Optics in"=w11541) -> ("error out"=w11539:errorcluster, "Optics out"=w11538:refnum<class "Opt_Selector.lvclass">)  [unwired: 7 in]
        n4830 = call "Write WPSEL.vi"("error in (no error)"=w11539, "Opt_Selector.lvclass"=w11538, "Instrument in"=w11536) -> ("error out"=w11532:errorcluster, "Instrument out"=w11531:refnum<class "Instrument.lvclass">)  [unwired: 7 in]
        n4831 = call "Read ASEL.vi"("error in (no error)"=w11532, "Instrument in"=w11531) -> ("error out"=w11549:errorcluster, "Opt_Selector.lvclass"=w11547:refnum<class "Opt_Selector.lvclass">, "Instrument out"=w11534:refnum<class "Instrument.lvclass">)  [unwired: 7 in]
        n4832 = call "Write target name.vi"("error in (no error)"=w11549, "target name"=w11439, "Optics in"=w11547) -> ("error out"=w11550:errorcluster, "Optics out"=w11546:refnum<class "Opt_Selector.lvclass">)  [unwired: 7 in]
        n4833 = Select(t="OFF", s=w11429, f=w11426) -> (s? t:f=w11427:string)
        n4834 = call "Write target.vi"("error in (no error)"=w11550, "target"=w11544, "Optics in"=w11546) -> ("error out"=w11551:errorcluster, "Optics out"=w11545:refnum<class "Opt_Selector.lvclass">)  [unwired: 7 in]
        n4835 = call "Write ASEL.vi"("error in (no error)"=w11551, "Opt_Selector.lvclass"=w11545, "Instrument in"=w11534) -> ("error out"=w11548:errorcluster, "Instrument out"=w11533:refnum<class "Instrument.lvclass">)  [unwired: 7 in]
        n4836 = call "Write Instrument.lvclass.vi"("error in (no error)"=w11548, "Instrument.lvclass"=w11533, "S4ACS_GUI in"=w11535) -> ("error out"=w11529:errorcluster, "S4ACS_GUI out"=w11530:refnum<class "S4GUI.lvclass">)  [unwired: 7 in]
        n4837 = call "Read Instrument.lvclass.vi"("error in (no error)"=w11529, "S4ACS_GUI in"=w11530) -> ("error out"=w11598:errorcluster, "Instrument.lvclass"=w11599:refnum<class "Instrument.lvclass">, "S4ACS_GUI out"=w11445:refnum<class "S4GUI.lvclass">)  [unwired: 7 in]
        n4838 = call "Read WPSEL.vi"("error in (no error)"=w11598, "Instrument in"=w11599) -> ("error out"=w11595:errorcluster, "Opt_Selector.lvclass"=w11597:refnum<class "Opt_Selector.lvclass">, "Instrument out"=w11589:refnum<class "Instrument.lvclass">)  [unwired: 7 in]
        n4839 = call-dynamic "Read State Machine.vi"("error in (no error)"=w11595, "Device in"=w11597) -> ("error out"=w11594:errorcluster, "State Machine.lvclass"=w11587:refnum<class "State Machine.lvclass">, "Device out"=w11591:refnum<class "Opt_Selector.lvclass">)  [unwired: 7 in]
        n4840 = call "Next State.vi"("error in (no error)"=w11594, "New_State"=1, "State Machine in"=w11587) -> ("error out"=w11593:errorcluster, "State Machine out"=w11592:refnum<class "State Machine.lvclass">)  [unwired: 7 in]
        n4841 = call-dynamic "Write State Machine.vi"("error in (no error)"=w11593, "State Machine.lvclass"=w11592, "Device in"=w11591) -> ("error out"=w11588:errorcluster, "Device out"=w11590:refnum<class "Opt_Selector.lvclass">)  [unwired: 7 in]
        n4842 = call "Write WPSEL.vi"("error in (no error)"=w11588, "Opt_Selector.lvclass"=w11590, "Instrument in"=w11589) -> ("error out"=w11579:errorcluster, "Instrument out"=w11578:refnum<class "Instrument.lvclass">)  [unwired: 7 in]
        n4843 = call "Read ASEL.vi"("error in (no error)"=w11579, "Instrument in"=w11578) -> ("error out"=w11585:errorcluster, "Opt_Selector.lvclass"=w11576:refnum<class "Opt_Selector.lvclass">, "Instrument out"=w11577:refnum<class "Instrument.lvclass">)  [unwired: 7 in]
        n4844 = call-dynamic "Read State Machine.vi"("error in (no error)"=w11585, "Device in"=w11576) -> ("error out"=w11584:errorcluster, "State Machine.lvclass"=w11580:refnum<class "State Machine.lvclass">, "Device out"=w11575:refnum<class "Opt_Selector.lvclass">)  [unwired: 7 in]
        n4845 = call "Next State.vi"("error in (no error)"=w11584, "New_State"=1, "State Machine in"=w11580) -> ("error out"=w11583:errorcluster, "State Machine out"=w11582:refnum<class "State Machine.lvclass">)  [unwired: 7 in]
        n4846 = call-dynamic "Write State Machine.vi"("error in (no error)"=w11583, "State Machine.lvclass"=w11582, "Device in"=w11575) -> ("error out"=w11581:errorcluster, "Device out"=w11574:refnum<class "Opt_Selector.lvclass">)  [unwired: 7 in]
        n4847 = Concatenate Strings("SET WAVEPLATE:  WPSEL=" ("string"), w11424, " CALW=" ("string"), w11427) -> (w11437:string)
        n4848 = call "Write ASEL.vi"("error in (no error)"=w11581, "Opt_Selector.lvclass"=w11574, "Instrument in"=w11577) -> ("error out"=w11561:errorcluster, "Instrument out"=w11563:refnum<class "Instrument.lvclass">)  [unwired: 7 in]
        n4849 = call "Read CALW.vi"("error in (no error)"=w11561, "Instrument in"=w11563) -> ("error out"=w11571:errorcluster, "Opt_Selector.lvclass"=w11573:refnum<class "Opt_Selector.lvclass">, "Instrument out"=w11562:refnum<class "Instrument.lvclass">)  [unwired: 7 in]
        n4850 = call-dynamic "Read State Machine.vi"("error in (no error)"=w11571, "Device in"=w11573) -> ("error out"=w11570:errorcluster, "State Machine.lvclass"=w11564:refnum<class "State Machine.lvclass">, "Device out"=w11567:refnum<class "Opt_Selector.lvclass">)  [unwired: 7 in]
        n4851 = call "Next State.vi"("error in (no error)"=w11570, "New_State"=1, "State Machine in"=w11564) -> ("error out"=w11569:errorcluster, "State Machine out"=w11568:refnum<class "State Machine.lvclass">)  [unwired: 7 in]
        n4852 = call-dynamic "Write State Machine.vi"("error in (no error)"=w11569, "State Machine.lvclass"=w11568, "Device in"=w11567) -> ("error out"=w11565:errorcluster, "Device out"=w11566:refnum<class "Opt_Selector.lvclass">)  [unwired: 7 in]
        n4853 = property on="Lambda Selector" class="Ring (strict)"() -> ("RingText.Text"=w11560:string)  [unwired: 2 in, 2 out]
        n4854 = call "Write CALW.vi"("error in (no error)"=w11565, "Opt_Selector.lvclass"=w11566, "Instrument in"=w11562) -> ("error out"=w11444:errorcluster, "Instrument out"=w11559:refnum<class "Instrument.lvclass">)  [unwired: 7 in]
        n4855 = call-dynamic "Read mode EXPOSE.vi"("error in (no error)"=w11444, "S4GUI in"=w11445) -> ("error out"=w11443:errorcluster, "mode EXPOSE"=w11441:bool, "S4GUI out"=w11442:refnum<class "S4GUI.lvclass">)  [unwired: 7 in]
        n4856 = call-dynamic "Read sync.vi"("error in (no error)"=w11443, "S4ACS_GUI in"=w11442) -> ("error out"=w11461:errorcluster, "sync"=w11460:bool, "S4ACS_GUI out"=w11462:refnum<class "S4GUI.lvclass">)  [unwired: 7 in]
        n4857 = case shown="\"OFF\"" w11560 {
          selector: w11560 -> [w11807 _]
          tunnel: w11559 -> [w11811 w11829]
          tunnel: [w11810 w11829] -> w11558
          tunnel: [w11803 w11828] -> w11478
          tunnel: w11461 -> [w11809 w11828]
          tunnel: [w11800 w11824] -> w11473
          tunnel: w11460 -> [w11799 _]
          tunnel: w11441 -> [w11798 w11827]
          frame "OFF" {
            w11801 = u16 0 items=["OFF", "POLARIZER", "PINHOLE", "SHUTTER", "DEPOLARIZER"] ("Calibrator Selector 2")
            n4858 = call "Read CALW.vi"("error in (no error)"=w11809, "Instrument in"=w11811) -> ("error out"=w11814:errorcluster, "Opt_Selector.lvclass"=w11816:refnum<class "Opt_Selector.lvclass">, "Instrument out"=w11815:refnum<class "Instrument.lvclass">)  [unwired: 7 in]
            n4859 = call "Write target.vi"("error in (no error)"=w11814, "target"=0.0, "Optics in"=w11816) -> ("error out"=w11813:errorcluster, "Optics out"=w11817:refnum<class "Opt_Selector.lvclass">)  [unwired: 7 in]
            n4860 = call "Write target name.vi"("error in (no error)"=w11813, "target name"=w11807, "Optics in"=w11817) -> ("error out"=w11812:errorcluster, "Optics out"=w11818:refnum<class "Opt_Selector.lvclass">)  [unwired: 7 in]
            n4861 = call "Write CALW.vi"("error in (no error)"=w11812, "Opt_Selector.lvclass"=w11818, "Instrument in"=w11815) -> ("error out"=w11802:errorcluster, "Instrument out"=w11810:refnum<class "Instrument.lvclass">)  [unwired: 7 in]
            n4862 = property on="Calibrator Selector" class="Ring (strict)"(error in=w11802, "Value"=w11801, "DisabledEnum"=T12."Disabled and Grayed Out" ("Disabled")) -> (error out=w11804:errorcluster)  [unwired: 1 in, 1 out]
            n4863 = property on="Calibrator Selector" class="Ring (strict)"(error in=w11804, "RingText.Text"="OFF" ("Ring Text.Text")) -> (error out=w11803:errorcluster)  [unwired: 1 in, 1 out]
            n4864 = case shown="True" w11799 {
              tunnel: [u8 0 ("SHUTTER_MODE") w11821] -> w11800
              tunnel: w11798 -> [_ w11820]
              frame False {
                # "Fotom. & Async"
                # "Internal"
              }
              frame True {
                # "Ext. Start"
                # "Internal"
                # "Fotom. Sync. SEM exp mode"
                # "Fotom. Sync. COM exp mode"
